vi "arr_to_bool_collect.vi"(4 "index":i32, 5 "array":dbl[](array[numeric])) -> (0 "Boolean array[3]":bool, 1 "Boolean array[2]":bool, 2 "Boolean array[1]":bool, 3 "Boolean array[0]":bool)   [LabVIEW 2014]
doc: "This vi converts element of an indexed array element into the collection of bolean values. \n\n\n\nCreated by \nBalaji V \nfor the purpose of learning about functions of loops(while & for)\nand it is submitted to the makcontrols india pvt ltd for the purpose of verification"
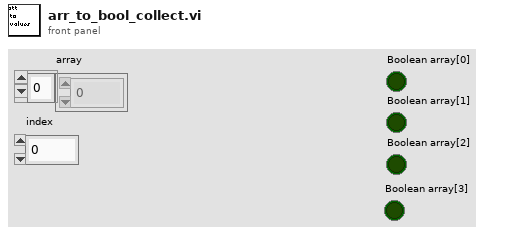
[diagram p1: front panel]
types:
  T1 = cluster{"Boolean array[0]":bool, "Boolean array[1]":bool, "Boolean array[2]":bool, "Boolean array[3]":bool, "Boolean array[4]":bool, "Boolean array[5]":bool, "Boolean array[6]":bool, "Boolean array[7]":bool, "Boolean array[8]":bool}
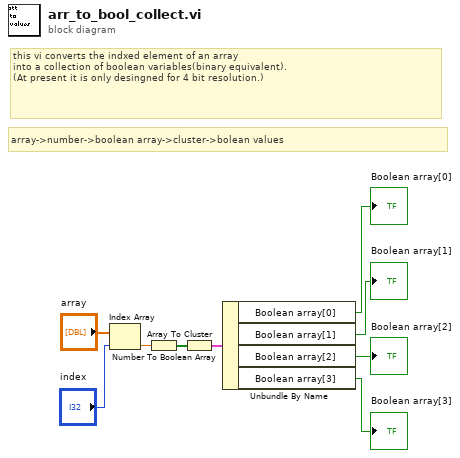
[diagram p0: block diagram]
diagram:
  # "array->number->boolean array->cluster->bolean values"
  # "this vi converts the indxed element of an array\ninto a collection of boolean variables(binary equivalent).\n(At present it is only desingned for 4 bit resolution.)"
  n1 = Index Array(array="array", index="index") -> (element=w9:dbl)
  n2 = Number To Boolean Array(number=w9) -> (Boolean array=w8:bool[])
  n3 = Array To Cluster(array=w8) -> (cluster=w7:T1)
  n4 = Unbundle By Name(w7) -> ("Boolean array[0]"=→"Boolean array[0]":bool, "Boolean array[1]"=→"Boolean array[1]":bool, "Boolean array[2]"=→"Boolean array[2]":bool, "Boolean array[3]"=→"Boolean array[3]":bool)
